vi "ConnectDetector_vi.vi"(8 "error in (no error)":errorcluster, 9 "Command":string, 10 "ON/OFF":bool, 11 "Control in":refnum<class "Control-Server.lvclass">) -> (0 "error out":errorcluster, 3 "Control out":refnum<class "Control-Server.lvclass">)   [LabVIEW 2015, in "Control-Server.lvclass"]
uses:
  Control-Server.lvclass
  dependecies/ControlsVIs/Clusters-def/Message types.ctl
  Control-Server.lvclass/Control-Server.ctl
  Detector/Detector.lvclass
  Message/Message.lvclass
  GeneralFunctionality/GeneralFunctionality.lvclass
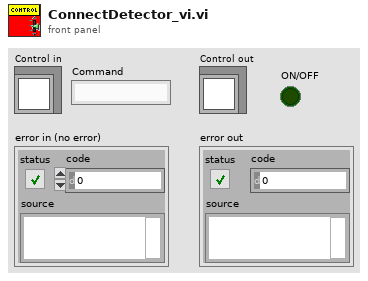
[diagram p1: front panel]
types:
  T1 = typedef "Message types.ctl" = string
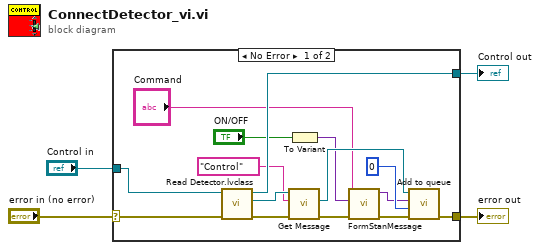
[diagram p0: block diagram]
diagram:
  n1 = case shown="No Error" "error in (no error)" {
    selector: "error in (no error)" -> [w18 w21]
    tunnel: "Control in" -> [w19 w20]
    tunnel: [w15 w20] -> w2
    tunnel: [w12 w21] -> w1
    frame No Error {
      n2 = call "Read Detector.lvclass.vi"("error in (no error)"=w18, "Control in"=w19) -> ("error out"=w16:errorcluster, "Detector.lvclass"=w17:refnum<class "Detector.lvclass">, "Control out"=w15:refnum<class "Control-Server.lvclass">)  [unwired: 7 in]
      n3 = call "Get Message.vi"("error in (no error)"=w16, "Message type"=T1 "Control", "GeneralFunctionality en entrée"=w17) -> ("error out"=w7:errorcluster, "Message.lvclass"=w10:refnum<class "Message.lvclass">)  [unwired: 6 in, 1 out]
      n4 = To Variant(anything="ON/OFF") -> (Variant=w6:variant)
      n5 = call "FormStanMessage.vi"("error in"=w7, "data"=w6, "Command"="Command") -> ("error out"=w8:errorcluster, "message"=w9:variant)  [unwired: 7 in]
      n6 = call "Add to queue.vi"("error in (no error)"=w8, "timeout in ms (-1)"=0, "Data"=w9, "Message in"=w10) -> ("error out"=w12:errorcluster)  [unwired: 6 in, 1 out]
    }
    frame Error {
    }
  }
  "Control out" <- w2
  "error out" <- w1
